vi "tm_datatoelectronframe.vi"(7 "Clip":bool, 8 "error in (no error)":errorcluster, 9 "Conversion Info":cluster{"coefficient":sgl, "offset":sgl}, 10 "Data Input":u16[][](array[numeric]), 11 "Handle in":u32) -> (0 "error out":errorcluster, 2 "Data Output":sgl[][](array[numeric]), 3 "Handle out":u32)   [LabVIEW 2012]
uses:
  tmcamcon.dll
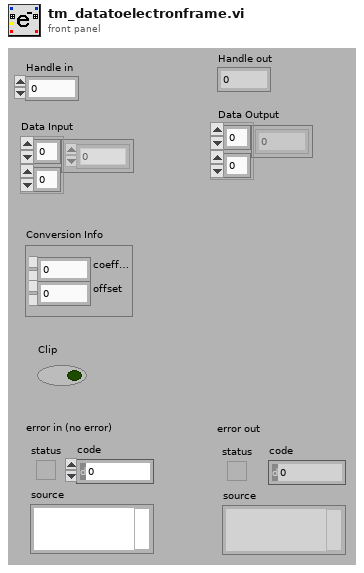
[diagram p1: front panel]
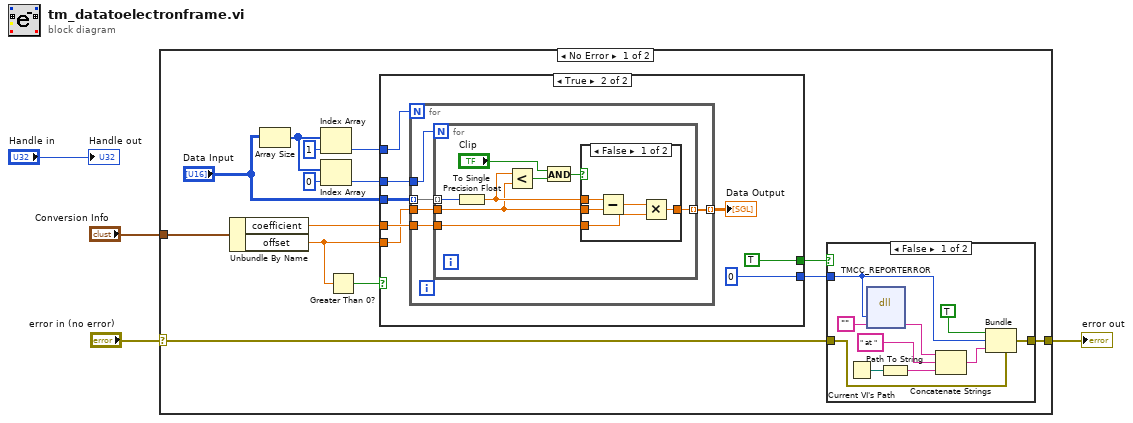
[diagram p0: block diagram]
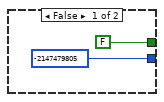
[diagram p2: hidden frame]
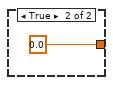
[diagram p3: hidden frame]
diagram:
  n1 = case shown="No Error" "error in (no error)" {
    selector: "error in (no error)" -> [w18 w59]
    tunnel: [w17 w59] -> w3
    tunnel: "Conversion Info" -> [w16 _]
    frame No Error {
      n2 = Unbundle By Name(w16) -> ("coefficient"=w14:sgl, "offset"=w13:sgl)
      n3 = Array Size(array="Data Input") -> (size(s)=w12:i32[])
      n4 = Index Array(array=w12, index=1) -> (element=w7:i32)
      n5 = Index Array(array=w12, index=0) -> (element=w8:i32)
      n6 = Greater Than 0?(x=w13) -> (x > 0?=w15:bool)
      n7 = case shown="True" w15 {
        tunnel: w14 -> [_ w27]
        tunnel: w13 -> [_ w21]
        tunnel: "Data Input" -> [_ w26]
        tunnel: w8 -> [_ w25]
        tunnel: w7 -> [_ w24]
        tunnel: [FALSE TRUE] -> w6
        tunnel: [-2147479805 0] -> w5
        frame False {
        }
        frame True {
          n8 = for {
            N: w24 -> [_]
            tunnel: w25 -> [w33]
            tunnel: w26 -> [w32] mode=indexing
            tunnel: w21 -> [w31]
            tunnel: w27 -> [w30]
            tunnel: [w29] -> w28 mode=indexing
            n9 = for {
              N: w33 -> [_]
              tunnel: w32 -> [w41] mode=indexing
              tunnel: w31 -> [w37]
              tunnel: w30 -> [w40]
              tunnel: [w39] -> w29 mode=indexing
              n10 = To Single Precision Float(number=w41) -> (single precision float=w38:sgl)
              n11 = Less?(x=w38, y=w37) -> (x < y?=w35:bool)
              n12 = And(x="Clip", y=w35) -> (x .and. y?=w36:bool)
              n13 = case shown="False" w36 {
                tunnel: w38 -> [w44 _]
                tunnel: w37 -> [w43 _]
                tunnel: w40 -> [w42 _]
                tunnel: [w45 sgl 0.0] -> w39
                frame False {
                  n14 = Subtract(x=w44, y=w43) -> (x-y=w46:sgl)
                  n15 = Multiply(x=w46, y=w42) -> (x*y=w45:sgl)
                }
                frame True {
                }
              }
            }
          }
          "Data Output" <- w28
        }
      }
      n16 = case shown="False" w6 {
        tunnel: w18 -> [w57 w58]
        tunnel: [w56 w58] -> w17
        tunnel: w5 -> [w50 _]
        frame False {
          n17 = Current VI's Path() -> (path=w55:path)
          n18 = dll-call lib="tmcamcon.dll" fn="TMCC_REPORTERROR"("error"=w50, "buf"="") -> ("buf"=w49:string)  [unwired: 5 in, 2 out]
          n19 = Path To String(path=w55) -> (string=w51:string)
          n20 = Concatenate Strings(w49, " at ", w51) -> (w54:string)
          n21 = Bundle(cluster=w57, "status"=TRUE, "code"=w50, "source"=w54) -> (w56:errorcluster)
        }
        frame True {
        }
      }
    }
    frame Error {
    }
  }
  "error out" <- w3
  "Handle out" <- "Handle in"
